vi "Event Camera.vi"() -> ()   [LabVIEW 2025]
panel:
  out "Image":T1(plugin-control)
  out "IP address":string
  in  "Stop recording":bool
  in  "Record":bool
  in  "Stop Preview":bool
  out "Output":string
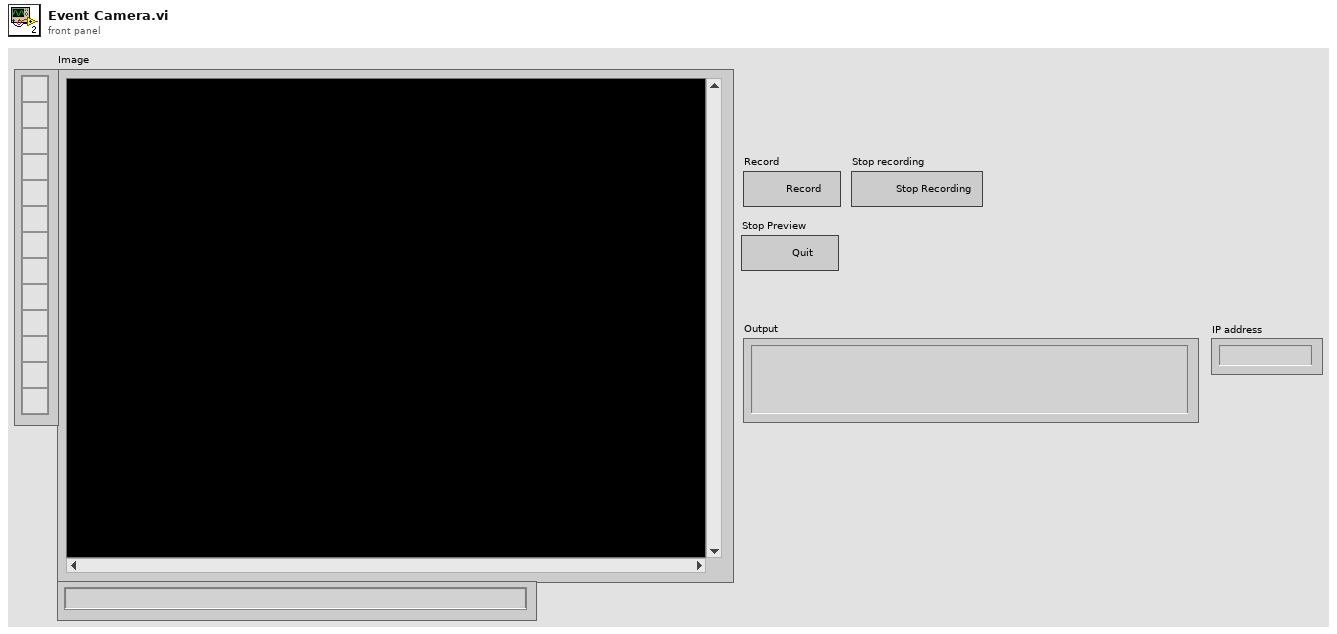
[diagram p1: front panel]
types:
  T1 = typedef "IMAQ Image.ctl" = refnum<image>
  T2 = enum16{"open", "replace", "create", "open or create", "replace or create", "replace or create with confirmation"}
  T3 = enum16{"big-endian, network order", "native, host order", "little-endian"}
  T4 = enum16{"Standard", "Buffered", "CRLF", "Immediate"}
  T5 = typedef "Image Type" = u32
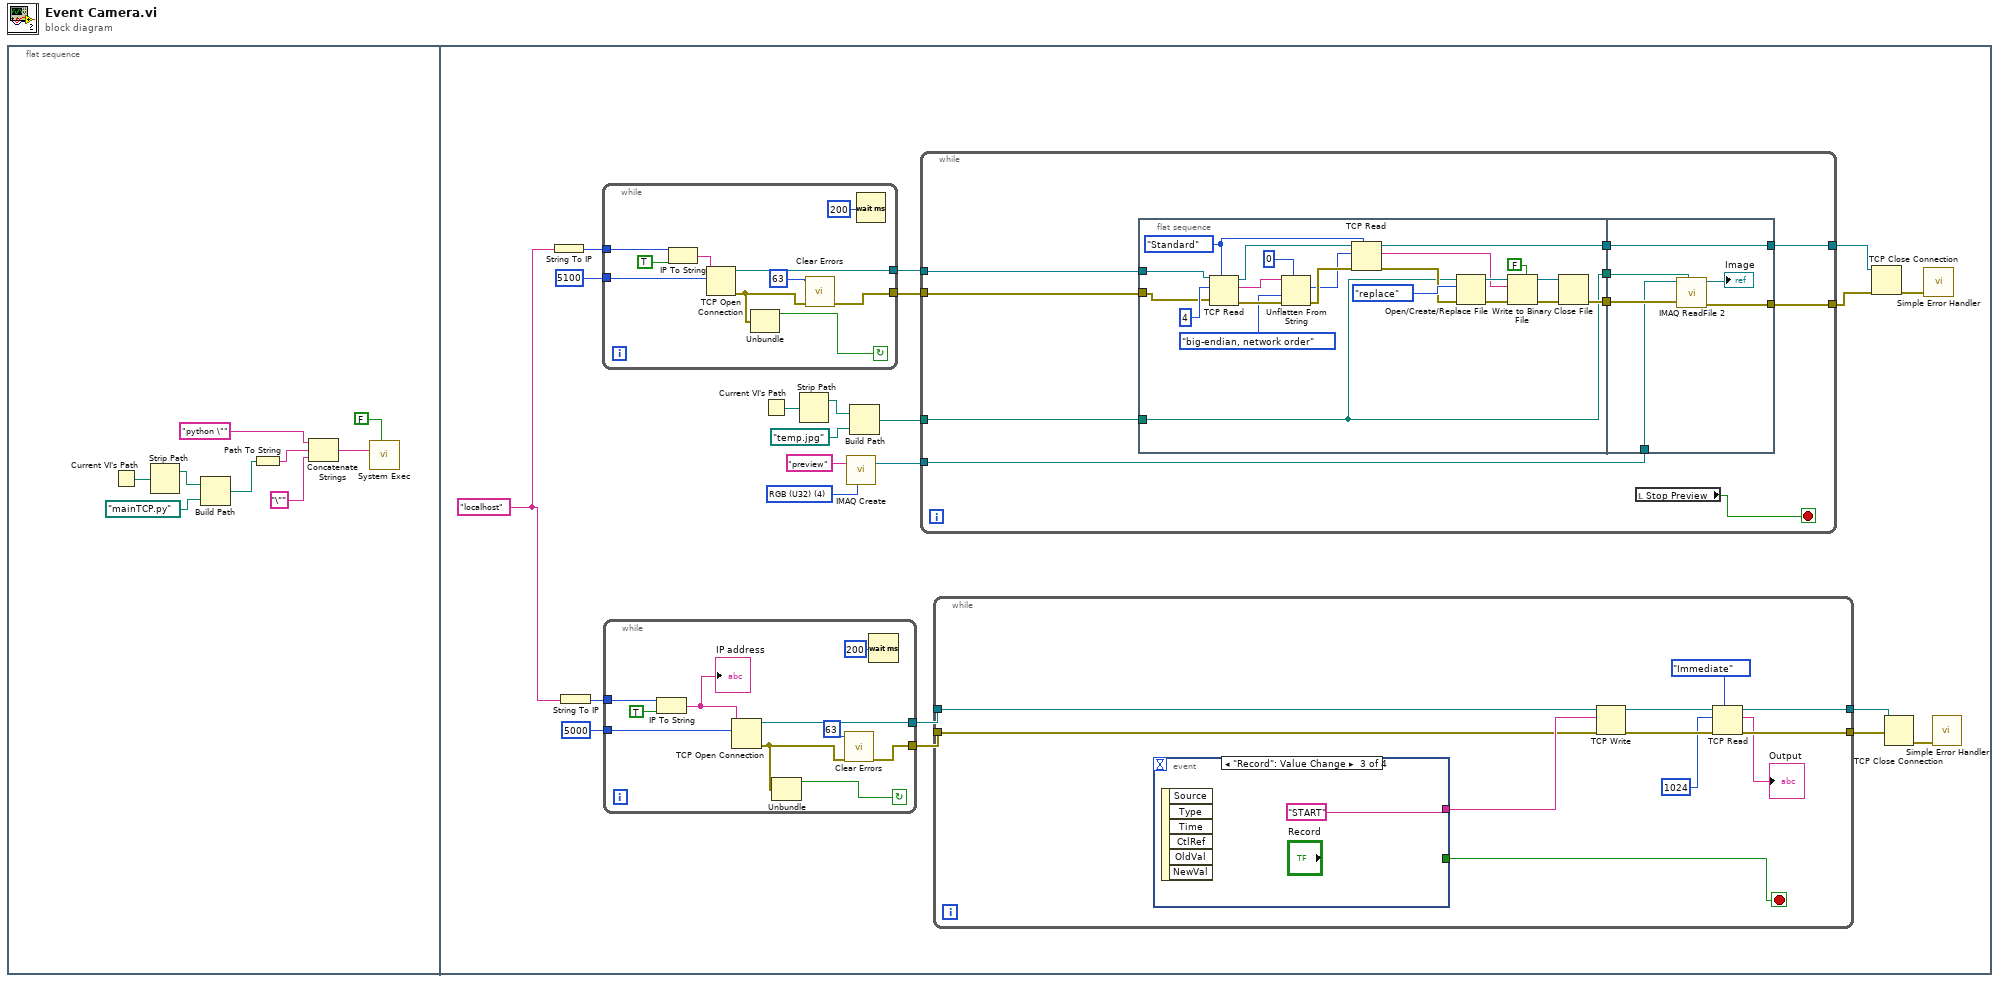
[diagram p0: block diagram]
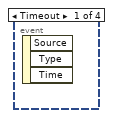
[diagram p2: hidden frame]
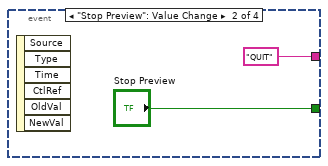
[diagram p3: hidden frame]
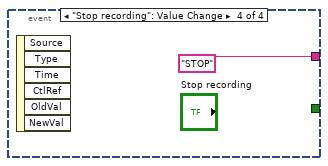
[diagram p4: hidden frame]
diagram:
  n1 = flat-sequence {
    frame #0 {
      n2 = Current VI's Path() -> (path=w4:path)
      n3 = Strip Path(path=w4) -> (stripped path=w5:path)  [unwired: 1 out]
      n4 = Build Path(base path=w5, name or relative path=path "mainTCP.py") -> (appended path=w2:path)
      n5 = Path To String(path=w2) -> (string=w8:string)
      n6 = Concatenate Strings("python \"" ("string"), w8, "\"" ("string")) -> (w7:string)
      n7 = call <vilib>:"System Exec.vi"("wait until completion? (T)"=FALSE, "command line"=w7) -> ()  [unwired: 6 in, 4 out]
    }
    frame #1 {
      w15 = T5 4 items=["Grayscale (U8)", "Grayscale (I16)", "Grayscale (SGL)", "Complex (CSG)", "RGB (U32)", "HSL (U32)", "RGB (U64)", "Grayscale (U16)"] ("Image Type")
      w10 = "localhost" ("name")
      n8 = String To IP(1:w10) -> (0:w14:u32)
      n9 = String To IP(1:w10) -> (0:w26:u32)
      n10 = while {
        tunnel: w14 -> [w41]
        tunnel: [w35] -> w13
        tunnel: [w39] -> w12
        tunnel: u16 5100 ("remote port or service name") -> [w37]
        stop <- w32 continue-if-true
        n11 = IP To String(1:TRUE ("dot notation? (F)"), 2:w41) -> (0:w40:string)
        n12 = TCP Open Connection(address=w40, remote port or service name=w37) -> (connection ID=w39:refnum<k5>, error out=w36:errorcluster)  [unwired: 3 in]
        n13 = Unbundle(w36) -> ("status"=w32:bool)  [unwired: 2 out]
        n14 = call <vilib>:"Clear Errors.vi"("error in (no error)"=w36, "specific error code to clear (0: all)"=63) -> ("error out"=w35:errorcluster)  [unwired: 4 in, 1 out]
        n15 = Wait (ms)(milliseconds to wait=u32 200) -> ()  [unwired: 1 out]
      }
      n16 = while {
        tunnel: [w83] -> w28
        tunnel: [w89] -> w27
        tunnel: w26 -> [w87]
        tunnel: u16 5000 ("remote port or service name") -> [w85]
        stop <- w80 continue-if-true
        n17 = IP To String(1:TRUE ("dot notation? (F)"), 2:w87) -> (0:w88:string)
        "IP address" <- w88
        n18 = TCP Open Connection(address=w88, remote port or service name=w85) -> (connection ID=w89:refnum<k5>, error out=w84:errorcluster)  [unwired: 3 in]
        n19 = Unbundle(w84) -> ("status"=w80:bool)  [unwired: 2 out]
        n20 = call <vilib>:"Clear Errors.vi"("error in (no error)"=w84, "specific error code to clear (0: all)"=63) -> ("error out"=w83:errorcluster)  [unwired: 4 in, 1 out]
        n21 = Wait (ms)(milliseconds to wait=u32 200) -> ()  [unwired: 1 out]
      }
      n22 = Current VI's Path() -> (path=w23:path)
      n23 = Strip Path(path=w23) -> (stripped path=w24:path)  [unwired: 1 out]
      n24 = call "IMAQ Create"("Image Name"="preview", "Image Type"=w15) -> ("New Image"=w19:T1)  [unwired: 3 in, 1 out]
      n25 = Build Path(base path=w24, name or relative path=path "temp.jpg") -> (appended path=w22:path)
      n26 = while {
        tunnel: w19 -> [w46]
        tunnel: [w47] -> w20
        tunnel: [w51] -> w21
        tunnel: w22 -> [w49]
        tunnel: w13 -> [w44]
        tunnel: w12 -> [w43]
        stop <- w42 stop-if-true
        n27 = flat-sequence {
          tunnel: w49 -> [w55]
          tunnel: [w57] -> w50
          tunnel: [w56] -> w48
          tunnel: [w55] -> w45
          tunnel: w44 -> [w53]
          tunnel: w43 -> [w52]
          tunnel: [w79] -> w51
          tunnel: w50 -> [w79]
          tunnel: w48 -> [w78]
          tunnel: [w77] -> w47
          tunnel: w46 -> [w76]
          tunnel: w45 -> [w75]
          frame #0 {
            w66 = T4."Standard" ("mode (standard)")
            n28 = TCP Read(connection ID=w52, bytes to read=4, error in (no error)=w53, 7:w66) -> (connection ID out=w69:refnum<k5>, data out=w54:string, error out=w72:errorcluster)  [unwired: 1 in]
            n29 = Unflatten From String(type=0, binary string=w54, byte order (0:big-endian, network order)=T3."big-endian, network order", error in (no error)=w72) -> (value=w67:i32, error out=w68:errorcluster)  [unwired: 1 in, 1 out]
            n30 = TCP Read(connection ID=w69, bytes to read=w67, error in (no error)=w68, 7:w66) -> (connection ID out=w57:refnum<k5>, data out=w62:string, error out=w64:errorcluster)  [unwired: 1 in]
            n31 = Open/Create/Replace File(file path (use dialog)=w55, error in=w64, operation (0:open)=T2."replace") -> (refnum out=w63:refnum<file>, error out=w60:errorcluster)  [unwired: 3 in, 1 out]
            n32 = Write to Binary File(file (use dialog)=w63, data=w62, error in=w60, 5:FALSE ("prepend array or string size? (T)")) -> (refnum out=w58:refnum<file>, error out=w59:errorcluster)  [unwired: 2 in, 1 out]
            n33 = Close File(refnum=w58, error in=w59) -> (error out=w56:errorcluster)  [unwired: 1 out]
          }
          frame #1 {
            n34 = call "IMAQ ReadFile 2"("File Path"=w75, "error in (no error)"=w78, "Image"=w76) -> ("error out"=w77:errorcluster, "Image Out"=→"Image":T1)  [unwired: 4 in, 3 out]
          }
        }
        n35 = local read "Stop Preview"() -> (w42:bool)
      }
      n36 = while {
        tunnel: [w99] -> w29
        tunnel: [w97] -> w30
        tunnel: w28 -> [w95]
        tunnel: w27 -> [w94]
        stop <- w90 stop-if-true
        n37 = event shown="[2] \"Record\": Value Change" {
          selector: _ -> [_ _ _ _]
          dyn-events: _ -> [_ _ _ _]
          timeout: _ -> [_ _ _ _]
          tunnel: [_ "QUIT" "START" "STOP"] -> w96
          tunnel: [_ "Stop Preview" _ _] -> w90
          event Timeout {
            n38 = event-data() -> ()  [unwired: 1 in, 3 out]
          }
          event "Stop Preview": Value Change {
            n39 = event-data() -> ()  [unwired: 1 in, 6 out]
          }
          event "Record": Value Change {
            n40 = event-data() -> ()  [unwired: 1 in, 6 out]
          }
          event "Stop recording": Value Change {
            n41 = event-data() -> ()  [unwired: 1 in, 6 out]
          }
        }
        n42 = TCP Write(connection ID=w94, data in=w96, error in (no error)=w95) -> (connection ID out=w98:refnum<k5>, error out=w100:errorcluster)  [unwired: 1 in, 1 out]
        n43 = TCP Read(connection ID=w98, bytes to read=1024, error in (no error)=w100, 7:T4."Immediate" ("mode (standard)")) -> (connection ID out=w97:refnum<k5>, data out=→"Output":string, error out=w99:errorcluster)  [unwired: 1 in]
      }
      n44 = TCP Close Connection(connection ID=w21, error in (no error)=w20) -> (error out=w18:errorcluster)  [unwired: 1 in, 1 out]
      n45 = TCP Close Connection(connection ID=w30, error in (no error)=w29) -> (error out=w31:errorcluster)  [unwired: 1 in, 1 out]
      n46 = call <vilib>:"Simple Error Handler.vi"("error in (no error)"=w18) -> ()  [unwired: 4 in, 5 out]
      n47 = call <vilib>:"Simple Error Handler.vi"("error in (no error)"=w31) -> ()  [unwired: 4 in, 5 out]
    }
  }
